vi "viTester.vi"   [LabVIEW 2014, in "G CLI VI Tester.lvlib"]
uses:
  G CLI VI Tester.lvlib
  <vilib>/Wiresmith Technology/G CLI/Argument Parser/Option Class/Option Configuration.ctl
  <vilib>/Wiresmith Technology/G CLI/Argument Parser/Option Class/Argument Type.ctl
  <vilib>/addons/_JKI Toolkits/VI Tester/TextTestRunner.llb/TextTestRunner.lvclass
  <vilib>/addons/_JKI.lib/_jki_lib_vi_tester_junit_xml_results.llb/TextTestRunner.JUnitXML.lvclass
  <vilib>/addons/_JKI Toolkits/VI Tester/VI Tester API.llb/Run Tests (Path).vi
  <vilib>/Wiresmith Technology/G CLI/CLI Class/CLI.lvclass
  <vilib>/Wiresmith Technology/G CLI/Argument Parser/Option Set Class/Option Set.lvclass
  <vilib>/Wiresmith Technology/G CLI/Argument Parser/Option Class/Option.lvclass
  <vilib>/addons/_JKI Toolkits/VI Tester/VI Tester API.llb/VI Tester API.lvlib
types:
  T1 = typedef "Option Parser.lvlib/Option.lvclass/Option Configuration.ctl" = cluster{"Option Type":T2, "Option Labels":string[], "Key":string, "Description":string, "Required":bool, "Default Value":string}
  T2 = typedef "Option Parser.lvlib/Option.lvclass/Argument Type.ctl" = enum16{"flag", "value"}
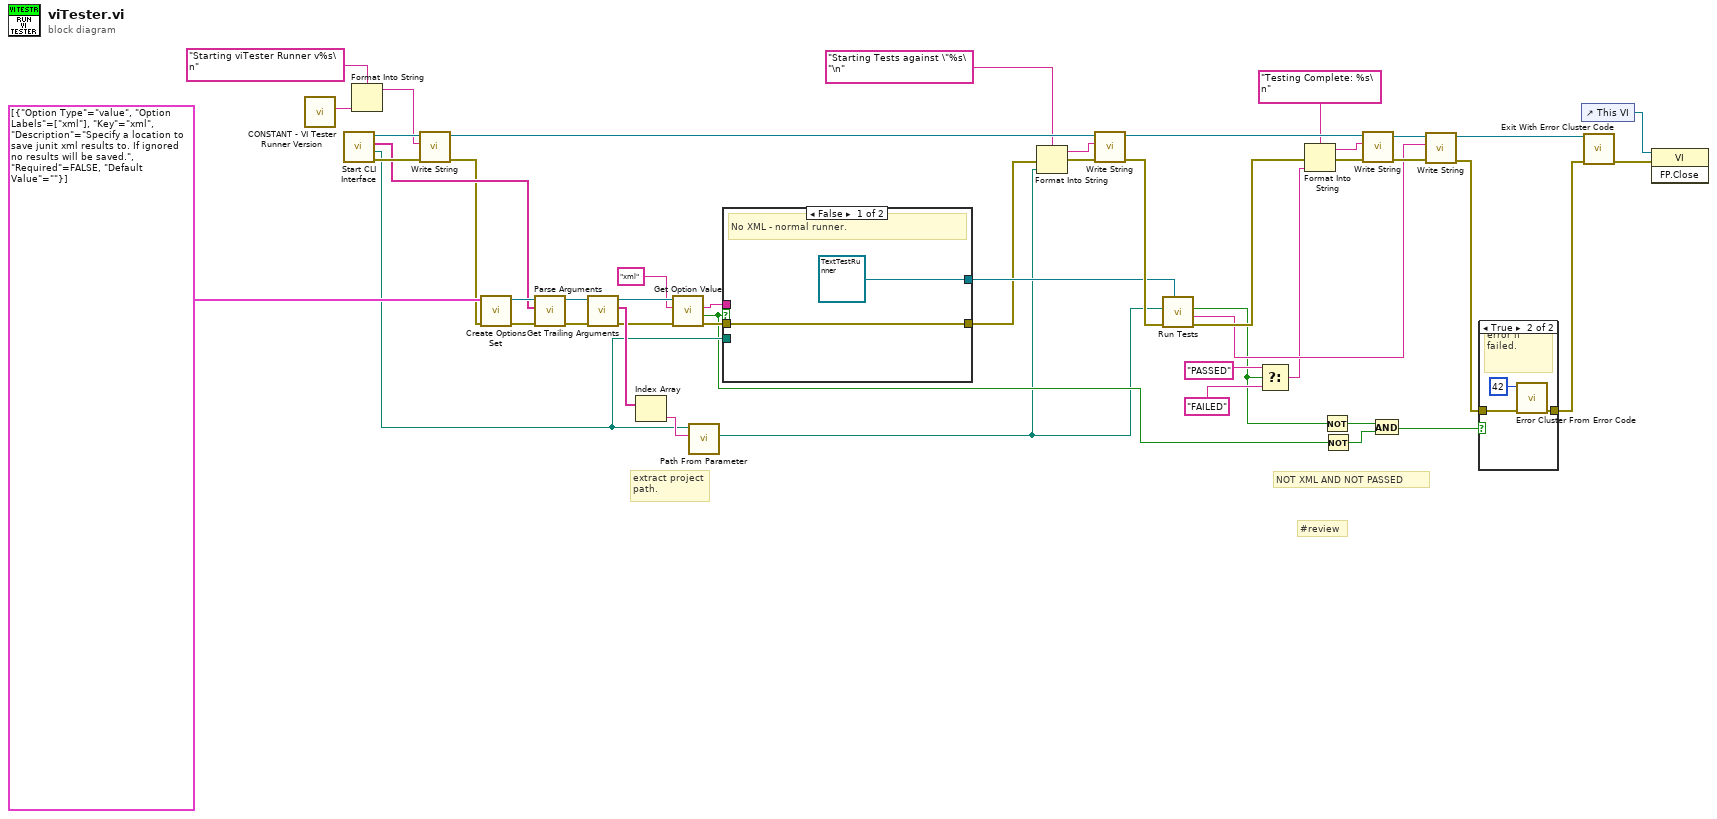
[diagram p0: block diagram]
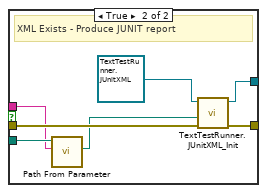
[diagram p3: hidden frame]
diagram:
  # "#review"
  # "NOT XML AND NOT PASSED"
  # "extract project\npath."
  n1 = call "CONSTANT - VI Tester Runner Version.vi"() -> ("Version"=w29:string)  [unwired: 11 in]
  n2 = call <vilib>:"Start CLI Interface.vi"() -> ("error out"=w48:errorcluster, "Working Directory"=w23:path, "Custom Parameters"=w45:string[], "CLI out"=w35:refnum<class "CLI.lvclass">)  [unwired: 8 in]
  n3 = Format Into String(format string="Starting viTester Runner v%s\n", w29) -> (resulting string=w32:string)  [unwired: 2 in, 1 out]
  n4 = call <vilib>:"Write String.vi"("error in (no error)"=w48, "Text to Write"=w32, "CLI in"=w35) -> ("error out"=w36:errorcluster, "CLI out"=w34:refnum<class "CLI.lvclass">)  [unwired: 7 in]
  n5 = call <vilib>:"Create Options Set.vi"("error in (no error)"=w36, "Options"=T1[] [{"Option Type"=enum."value", "Option Labels"=["xml"], "Key"="xml", "Description"="Specify a location to save junit xml results to. If ignored no results will be saved.", "Required"=FALSE, "Default Value"=""}]) -> ("error out"=w46:errorcluster, "Option Set out"=w47:refnum<class "Option Set.lvclass">)  [unwired: 8 in]
  n6 = call <vilib>:"Parse Arguments.vi"("error in (no error)"=w46, "Arguments"=w45, "Option Set in"=w47) -> ("error out"=w43:errorcluster, "Option Set out"=w44:refnum<class "Option Set.lvclass">)  [unwired: 5 in, 2 out]
  n7 = call <vilib>:"Get Trailing Arguments.vi"("error in (no error)"=w43, "Option Set in"=w44) -> ("error out"=w40:errorcluster, "Arguments"=w42:string[], "Option Set out"=w39:refnum<class "Option Set.lvclass">)  [unwired: 7 in]
  n8 = Index Array(array=w42) -> (element=w41:string)  [unwired: 1 in]
  n9 = call <vilib>:"Get Option Value.vi"("error in (no error)"=w40, "Option Key"="xml", "Option Set in"=w39) -> ("error out"=w25:errorcluster, "Set"=w6:bool, "Value"=w22:string)  [unwired: 5 in, 1 out]
  n10 = call <vilib>:"Path From Parameter.vi"("Path Parameter"=w41, "Working Directory"=w23) -> ("Full Path"=w1:path)  [unwired: 9 in]
  n11 = case shown="False" w6 {
    tunnel: [refnum<class "TextTestRunner.lvclass"> refnum ("TextTestRunner in") w55] -> w26
    tunnel: w25 -> [w50 w57]
    tunnel: [w50 w58] -> w24
    tunnel: w23 -> [_ w54]
    tunnel: w22 -> [_ w53]
    frame False {
      # "No XML - normal runner."
    }
    frame True {
      # "XML Exists - Produce JUNIT report"
      n12 = call <vilib>:"Path From Parameter.vi"("Path Parameter"=w53, "Working Directory"=w54) -> ("Full Path"=w52:path)  [unwired: 9 in]
      n13 = call <vilib>:"TextTestRunner.JUnitXML_Init.vi"("error in (no error)"=w57, "Report Path"=w52, "TextTestRunner in"=refnum<class "TextTestRunner.JUnitXML.lvclass"> refnum ("TextTestRunner.Ant.lvclass")) -> ("error out"=w58:errorcluster, "TextTestRunner out"=w55:refnum<class "TextTestRunner.JUnitXML.lvclass">)  [unwired: 7 in]
    }
  }
  n14 = Format Into String(format string="Starting Tests against \"%s\"\n" ("Text to Write"), error in=w24, w1) -> (resulting string=w3:string, error out=w4:errorcluster)  [unwired: 1 in]
  n15 = call <vilib>:"Write String.vi"("error in (no error)"=w4, "Text to Write"=w3, "CLI in"=w34) -> ("error out"=w28:errorcluster, "CLI out"=w37:refnum<class "CLI.lvclass">)  [unwired: 7 in]
  n16 = call-poly <vilib>:"Run Tests.vi"("TextTestRunner in"=w26, "error in (no error)"=w28, "Test Path"=w1) -> ("error out"=w27:errorcluster, "test details"=w17:string, "successful?"=w9:bool)  [unwired: 6 in]
  n17 = Select(t="PASSED", s=w9, f="FAILED") -> (s? t:f=w13:string)
  n18 = Format Into String(format string="Testing Complete: %s\n" ("Text to Write"), error in=w27, w13) -> (resulting string=w14:string, error out=w16:errorcluster)  [unwired: 1 in]
  n19 = Not(x=w9) -> (.not. x?=w7:bool)
  n20 = Not(x=w6) -> (.not. x?=w5:bool)
  n21 = call <vilib>:"Write String.vi"("error in (no error)"=w16, "Text to Write"=w14, "CLI in"=w37) -> ("error out"=w18:errorcluster, "CLI out"=w19:refnum<class "CLI.lvclass">)  [unwired: 7 in]
  n22 = And(x=w7, y=w5) -> (x .and. y?=w8:bool)
  n23 = call <vilib>:"Write String.vi"("error in (no error)"=w18, "Text to Write"=w17, "CLI in"=w19) -> ("error out"=w20:errorcluster, "CLI out"=w21:refnum<class "CLI.lvclass">)  [unwired: 7 in]
  n24 = case shown="True" w8 {
    tunnel: w20 -> [w59 w62]
    tunnel: [w59 w61] -> w10
    frame False {
    }
    frame True {
      # "error if failed."
      n25 = call <vilib>:"Error Cluster From Error Code.vi"("error in (no error)"=w62, "error code (0)"=42) -> ("error out"=w61:errorcluster)  [unwired: 7 in]
    }
  }
  n26 = control-ref of="This VI"() -> (w31:refnum<vi>)
  n27 = call <vilib>:"Exit With Error Cluster Code.vi"("error in (no error)"=w10, "CLI in"=w21) -> ("error out"=w30:errorcluster)  [unwired: 9 in]
  n28 = invoke class="VI" method="FP.Close"(reference=w31, error in=w30) -> ()  [unwired: 1 in, 3 out]
